vi "String_to_Ch_names.vi"(0 "Spreadsheet string":string) -> (1 "Ch names":string[](array[string]), 2 "Title length (Bytes)":i32, 3 "Title Rows Found?":bool, 4 "String After names":string)   [LabVIEW 2016]
panel:
  out "Data length":i32
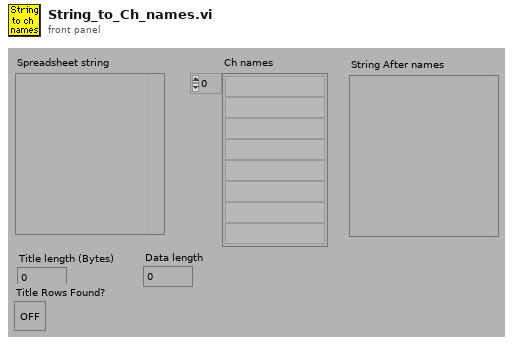
[diagram p1: front panel]
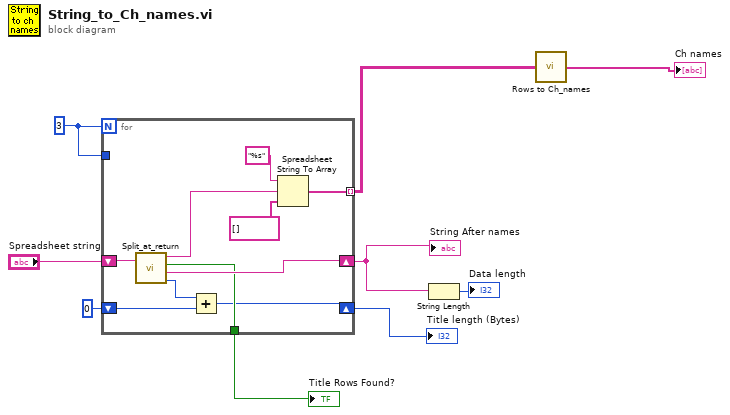
[diagram p0: block diagram]
diagram:
  w9 = 3
  n1 = for {
    N: w9 -> [_]
    shift-right: [w15] -> w6
    shift-left: "Spreadsheet string" -> [w16]
    tunnel: w9 -> [_]
    tunnel: [w14] -> w5
    tunnel: [w13] -> w4 mode=indexing
    shift-right: [w10] -> w1
    shift-left: 0 -> [w11]
    n2 = call "Split_at_return.vi"("String"=w16) -> ("before substring"=w17:string, "Matched?"=w14:bool, "after substring"=w15:string, "offset past match"=w12:i32)  [unwired: 1 in]
    n3 = Add(x=w12, y=w11) -> (x+y=w10:i32)
    n4 = Spreadsheet String To Array(format string="%s", spreadsheet string=w17, array type (2D Dbl)=string[] []) -> (array=w13:string[])  [unwired: 1 out]
  }
  "Title length (Bytes)" <- w1
  "String After names" <- w6
  "Title Rows Found?" <- w5
  n5 = String Length(string=w6) -> (length=→"Data length":i32)
  n6 = call "Rows to Ch_names.vi"("array type (2D Dbl)"=w4) -> ("Array"=→"Ch names":string[])
